vi "Teardown.vi"(11 "jettl Event Actor in":refnum<class "jettl Event Actor.lvclass">) -> (3 "jettl Event Actor out":refnum<class "jettl Event Actor.lvclass">)   [LabVIEW 2021, in "jettl.lvlib" / "jettl Event Actor.lvlib" / "jettl Event Actor.lvclass"]
uses:
  jettl Event Actor.lvclass
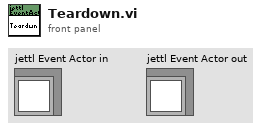
[diagram p1: front panel]
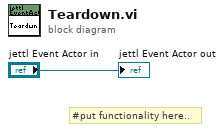
[diagram p0: block diagram]
diagram:
  # "#put functionality here.."
  "jettl Event Actor out" <- "jettl Event Actor in"
